vi "Remove.vi"() -> ()   [LabVIEW 2024, in "RefTypedCircularBuffer.Tests.Units.lvlib"]
uses:
  RefTypedCircularBuffer.Tests.Units.lvlib
  <vilib>/addons/_JKI Toolkits/Caraya/classes/Assert/Assert.lvclass
  <vilib>/addons/_JKI Toolkits/Caraya/classes/Test/Test.lvclass
  <vilib>/addons/_JKI Toolkits/Caraya/classes/Assert/Assert True.vi
  <vilib>/addons/_JKI Toolkits/Caraya/classes/Assert/Assert False.vi
  RefTypedCircularBuffer.lvclass
  TypedCircularBuffer/Type.ctl
  TypedCircularBuffer/TypedCircularBuffer.lvclass
panel:
  out "element":T1
  in  "expected":i32[](array[numeric])=[2, 3, 4, 5, 6, 7, 8, 9, 10]
  out "Flushed Buffer":T1[](array[typedef])
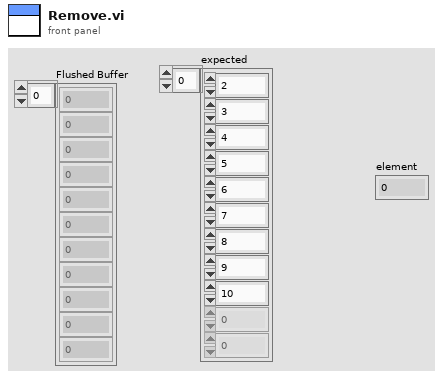
[diagram p1: front panel]
types:
  T1 = typedef "TypedCircularBuffer.lvclass/Type.ctl" = i32
  T2 = typedef "RefTypedCircularBuffer.lvclass/Type.ctl" = u8
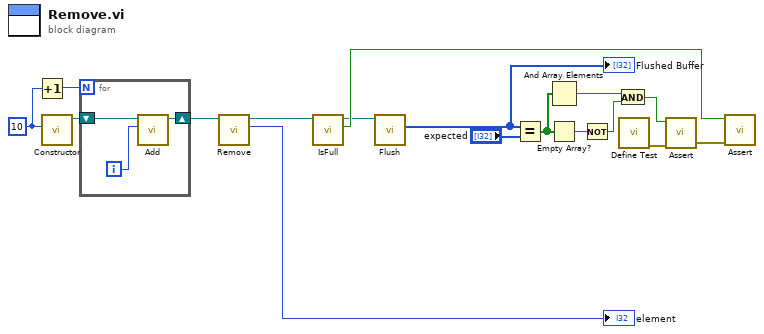
[diagram p0: block diagram]
diagram:
  w7 = u32 10 ("Capacity")
  n1 = Increment(x=w7) -> (x+1=w17:u32)
  n2 = call "Constructor.vi"("Capacity"=w7) -> ("TypedCircularBuffer out"=w8:refnum<class "RefTypedCircularBuffer.lvclass">)  [unwired: 10 in]
  n3 = for {
    N: w17 -> [_]
    shift-right: [w18] -> w6
    shift-left: w8 -> [w20]
    i -> [w19]
    n4 = call "Add.vi"("Element"=w19, "TypedCircularBuffer in"=w20) -> ("TypedCircularBuffer out"=w18:refnum<class "RefTypedCircularBuffer.lvclass">)  [unwired: 7 in, 2 out]
  }
  n5 = call "Remove.vi"("TypedCircularBuffer in"=w6) -> ("element"=→"element":T2, "TypedCircularBuffer out"=w4:refnum<class "RefTypedCircularBuffer.lvclass">)  [unwired: 8 in, 1 out]
  n6 = call "IsFull.vi"("TypedCircularBuffer in"=w4) -> ("Full?"=w3:bool, "TypedCircularBuffer out"=w2:refnum<class "RefTypedCircularBuffer.lvclass">)  [unwired: 9 in]
  n7 = call "Flush.vi"("TypedCircularBuffer in"=w2) -> ("Flushed Buffer"=w1:T2[])  [unwired: 9 in, 1 out]
  "Flushed Buffer" <- w1
  n8 = Equal?(x=w1, y="expected") -> (x = y?=w13:bool[])
  n9 = And Array Elements(Boolean array=w13) -> (logical AND=w16:bool)
  n10 = Empty Array?(array=w13) -> (empty?=w15:bool)
  n11 = Not(x=w15) -> (.not. x?=w14:bool)
  n12 = And(x=w16, y=w14) -> (x .and. y?=w12:bool)
  n13 = call <vilib>:"Define Test.vi"() -> ("error out"=w11:errorcluster)  [unwired: 10 in, 1 out]
  n14 = call-poly <vilib>:"Assert.vi"("error in (no error)"=w11, "True?"=w12) -> ("error out"=w9:errorcluster)  [unwired: 8 in, 1 out]
  n15 = call-poly <vilib>:"Assert.vi"("error in (no error)"=w9, "False?"=w3) -> ()  [unwired: 8 in, 2 out]
